vi "generate signal.vi"(8 "noise (rms)":dbl=0.1 format="%.2p", 9 "cluster 3":T1={"frequency"=1000.0, "amplitude"=5.0, "phase"=0.0}, 10 "cluster 2":T1={"frequency"=8000.0, "amplitude"=5.0, "phase"=0.0}, 11 "cluster":T1={"frequency"=1500.0, "amplitude"=3.0, "phase"=0.0}) -> (3 "Waveform Graph 5":waveform(dbl)(graph)={"t0"=timestamp(0.4 s since 1904-01-01), "dt"=1e-05, "Y"=array[10000 elements]})   [LabVIEW 2015]
uses:
  <vilib>/measure/NI_MABase.lvlib
panel:
  in  "stop":bool
  out "Waveform Graph 4":waveform(dbl)(graph)={"t0"=timestamp(0.4 s since 1904-01-01), "dt"=1e-05, "Y"=array[10000 elements]}
  out "Waveform Graph 3":waveform(dbl)(graph)={"t0"=timestamp(0.4 s since 1904-01-01), "dt"=1e-05, "Y"=array[10000 elements]}
  out "Waveform Graph 2":waveform(dbl)(graph)={"t0"=timestamp(0.4 s since 1904-01-01), "dt"=1e-05, "Y"=array[10000 elements]}
  out "Waveform Graph":waveform(dbl)(graph)={"t0"=timestamp(0.4 s since 1904-01-01), "dt"=1e-05, "Y"=array[10000 elements]}
  # "SIGNAL 1"
  # "GENERATED SIGNAL"
  # "SIGNAL 2"
  # "SIGNAL 3"
  # "NOISE"
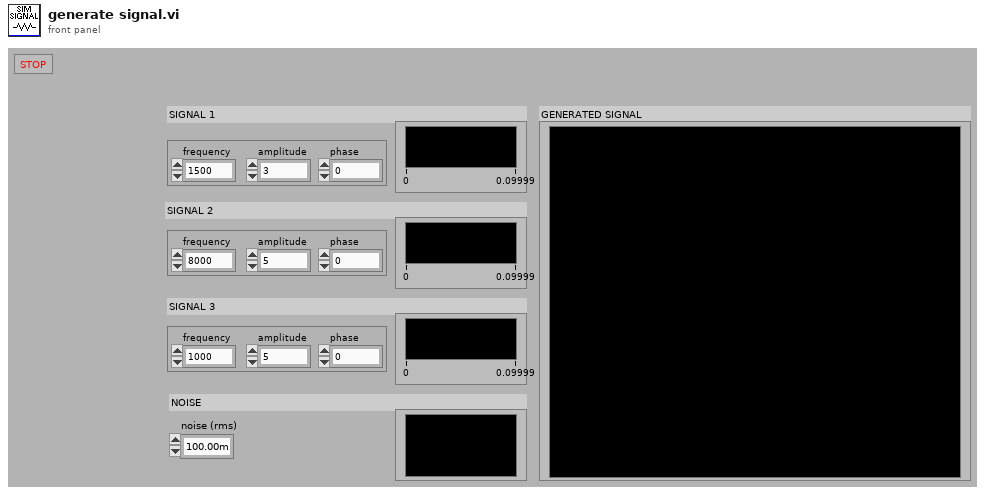
[diagram p1: front panel]
types:
  T1 = cluster{"frequency":dbl, "amplitude":dbl, "phase":dbl}
  T2 = cluster{"frequency":dbl, "amplitude":dbl, "phase":dbl}[]
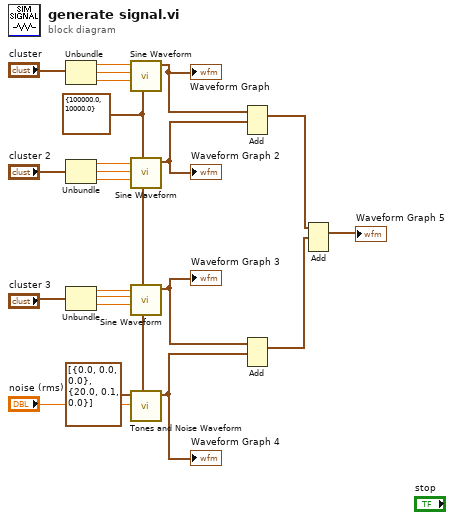
[diagram p0: block diagram]
diagram:
  w8 = cluster{"Fs":dbl, "#s":dbl} {"Fs"=100000.0, "#s"=10000.0} ("sampling info")
  n1 = Unbundle("cluster") -> ("frequency"=w14:dbl, "amplitude"=w13:dbl, "phase"=w12:dbl)
  n2 = Unbundle("cluster 2") -> ("frequency"=w11:dbl, "amplitude"=w10:dbl, "phase"=w9:dbl)
  n3 = Unbundle("cluster 3") -> ("frequency"=w1:dbl, "amplitude"=w7:dbl, "phase"=w6:dbl)
  n4 = call <vilib>:"Sine Waveform.vi"("sampling info"=w8, "phase"=w12, "amplitude"=w13, "frequency"=w14) -> ("signal out"=w19:waveform(dbl))  [unwired: 6 in, 1 out]
  "Waveform Graph" <- w19
  n5 = call <vilib>:"Sine Waveform.vi"("sampling info"=w8, "phase"=w9, "amplitude"=w10, "frequency"=w11) -> ("signal out"=w18:waveform(dbl))  [unwired: 6 in, 1 out]
  "Waveform Graph 2" <- w18
  n6 = call <vilib>:"Sine Waveform.vi"("sampling info"=w8, "phase"=w6, "amplitude"=w7, "frequency"=w1) -> ("signal out"=w16:waveform(dbl))  [unwired: 6 in, 1 out]
  "Waveform Graph 3" <- w16
  n7 = call <vilib>:"Tones and Noise Waveform.vi"("sampling info"=w8, "noise (rms)"="noise (rms)", "tones"=T2 [{"frequency"=0.0, "amplitude"=0.0, "phase"=0.0}, {"frequency"=20.0, "amplitude"=0.1, "phase"=0.0}]) -> ("signal out"=w17:waveform(dbl))  [unwired: 7 in, 1 out]
  "Waveform Graph 4" <- w17
  n8 = Add(1:w18, 2:w19) -> (0:w21:waveform(dbl))  [unwired: 1 in, 1 out]
  n9 = Add(1:w17, 2:w16) -> (0:w20:waveform(dbl))  [unwired: 1 in, 1 out]
  n10 = Add(1:w20, 2:w21) -> (0:→"Waveform Graph 5":waveform(dbl))  [unwired: 1 in, 1 out]
